vi "Parse Result Key.vi"(8 "error in (no error)":errorcluster, 9 "Ref Channel":i32, 10 "AI Channel":i32, 11 "Datatype":string) -> (0 "error out":errorcluster, 2 "Label":string, 3 "Key":string)   [LabVIEW 2019, in "Instrument.Lockin.lvclass"]
uses:
  Instrument.Lockin.lvclass
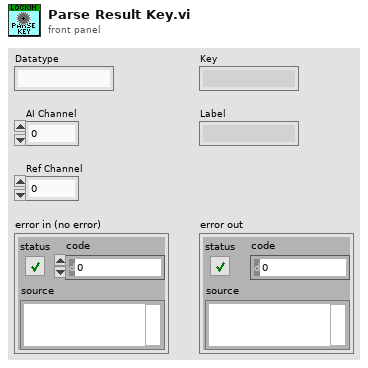
[diagram p1: front panel]
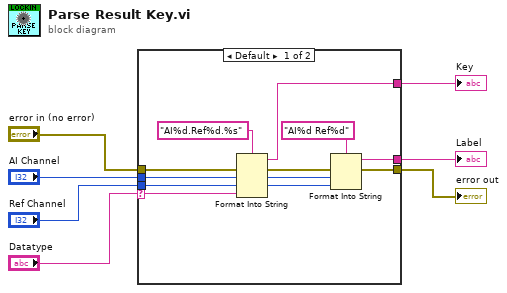
[diagram p0: block diagram]
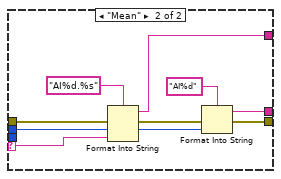
[diagram p2: hidden frame]
diagram:
  n1 = case shown="Default" "Datatype" {
    selector: "Datatype" -> [w8 w18]
    tunnel: "Ref Channel" -> [w9 _]
    tunnel: "AI Channel" -> [w17 w26]
    tunnel: [w16 w25] -> w6
    tunnel: "error in (no error)" -> [w15 w24]
    tunnel: [w13 w22] -> w4
    tunnel: [w11 w20] -> w3
    frame Default {
      n2 = Format Into String(format string="AI%d.Ref%d.%s", error in=w15, w17, w9, w8) -> (resulting string=w11:string, error out=w14:errorcluster)  [unwired: 1 in]
      n3 = Format Into String(format string="AI%d Ref%d", error in=w14, w17, w9) -> (resulting string=w13:string, error out=w16:errorcluster)  [unwired: 1 in]
    }
    frame "Mean" {
      n4 = Format Into String(format string="AI%d.%s", error in=w24, w26, w18) -> (resulting string=w20:string, error out=w23:errorcluster)  [unwired: 1 in]
      n5 = Format Into String(format string="AI%d", error in=w23, w26) -> (resulting string=w22:string, error out=w25:errorcluster)  [unwired: 1 in]
    }
  }
  "error out" <- w6
  "Label" <- w4
  "Key" <- w3
